vi "draw_extrapolated_lines.vi"(8 "error in (no error)":errorcluster, 11 "TrajectoryMH100122AODRAPS in":refnum<class "TrajectoryMH100122AODRAPS.lvclass">) -> (0 "error out":errorcluster, 3 "TrajectoryMH100122AODRAPS out":refnum<class "TrajectoryMH100122AODRAPS.lvclass">)   [LabVIEW 2010, in "TrajectoryMH100122AODRAPS.lvclass"]
uses:
  TrajectoryMH100122AODRAPS.lvclass
  roi_visualization_cluster.ctl
  common/xcontrols/XImage/XImage/overlays_cluster.ctl
  common/xcontrols/XImage/XImage/XImage.xctl
  TrajectoryMH100122AODRAPS.lvclass/TrajectoryMH100122AODRAPS.ctl
  class_data.vi
  <vilib>/Analysis/1siggen.llb/Ramp Pattern by Samples.vi
  <vilib>/Analysis/NI_AALBase.lvlib
panel:
  in  "zoom":dbl=100.0
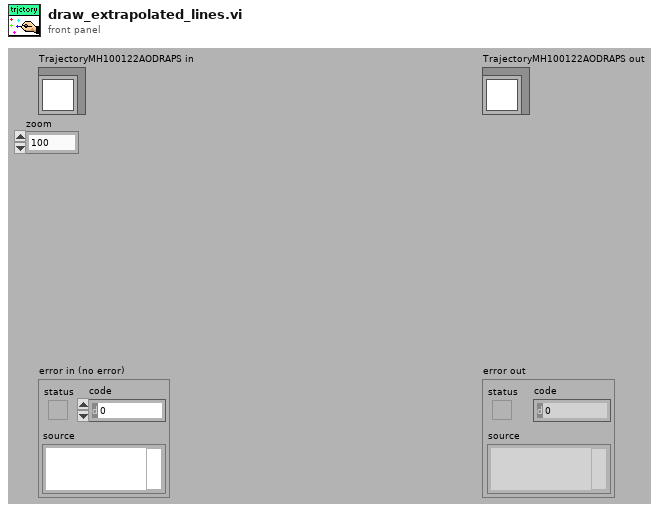
[diagram p1: front panel]
types:
  T1 = typedef "XImage.xctl/overlays_cluster.ctl" = cluster{"overlay array":cluster{i32[][]}[], "overlay name":string, "color (red)":u32, "overlay size":i32, "overlay type":enum16{"crosshair", "circle"}}
  T2 = typedef "TrajectoryMH100122AODRAPS.lvclass/roi_visualization_cluster.ctl" = cluster{"counter":i32, "type":u16, "activation":bool}
  T3 = cluster{"Global Rectangle":i32[], "Contours":cluster{"Contour Type":u32, "ROI Type":u32, "Points":i32[]}[]}[]
  T4 = cluster{"Contour Type":u32, "ROI Type":u32, "Points":i32[]}[]
  T5 = typedef "roi_visualization_cluster.ctl" = cluster{"counter":i32, "type":u16, "activation":bool}
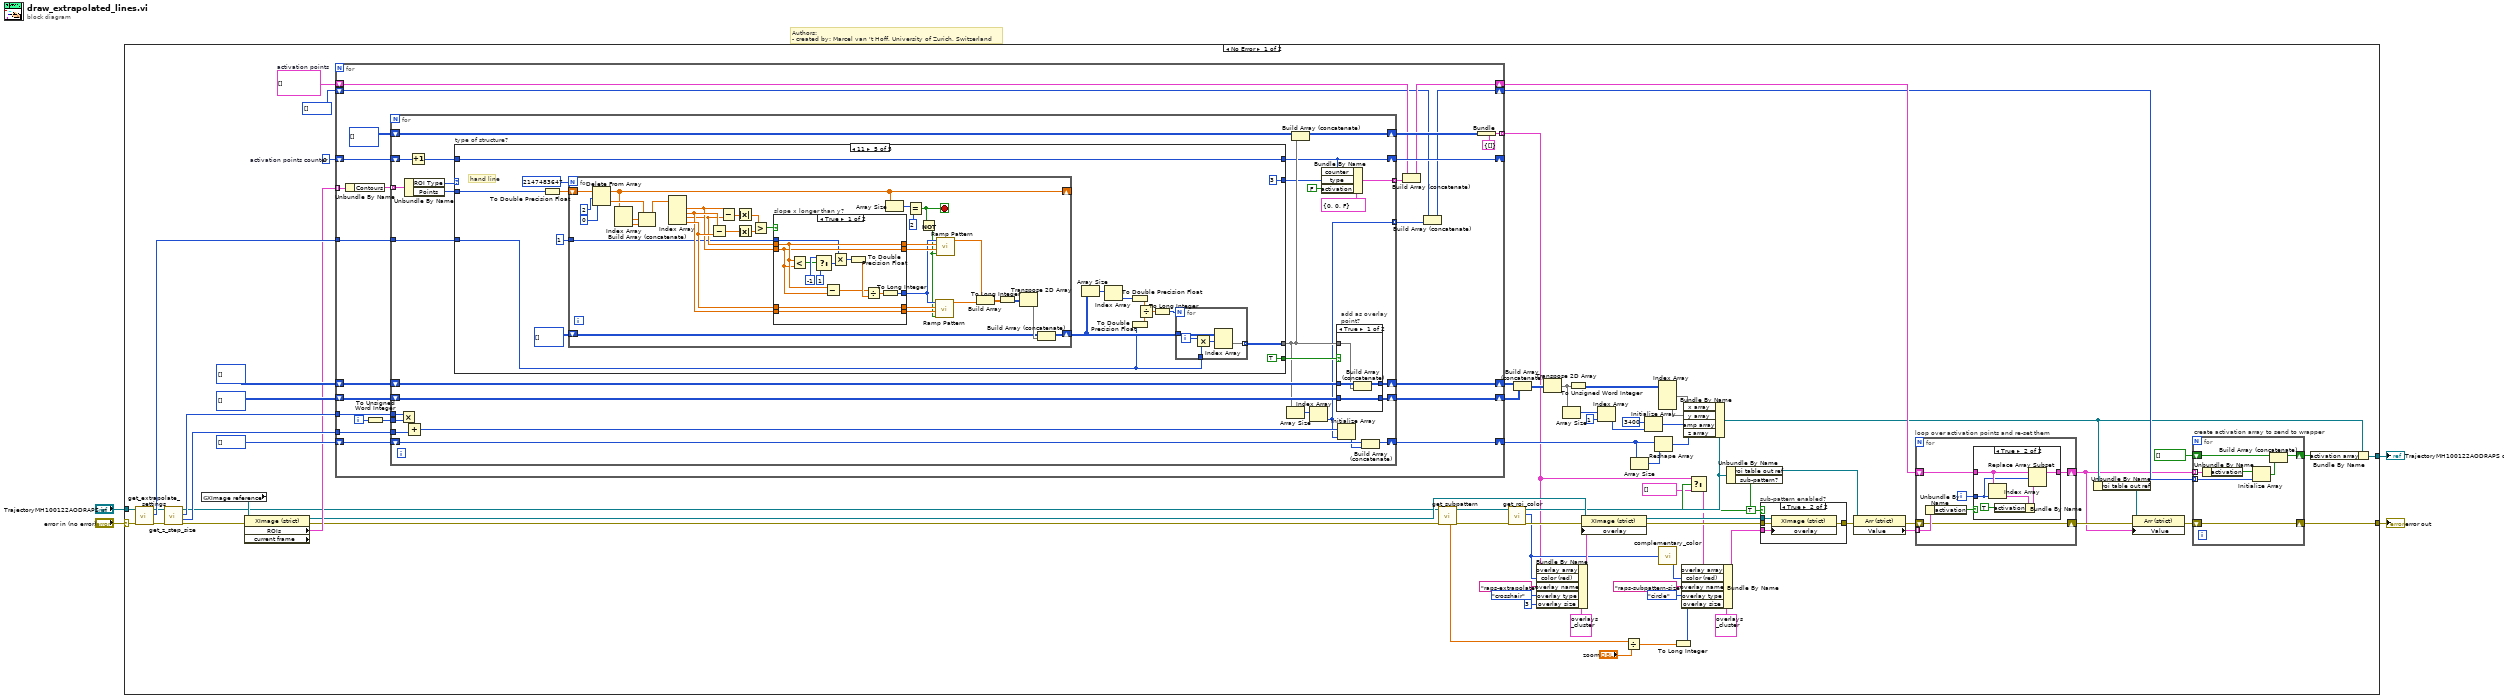
[diagram p0: block diagram]
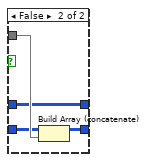
[diagram p4: hidden frame]
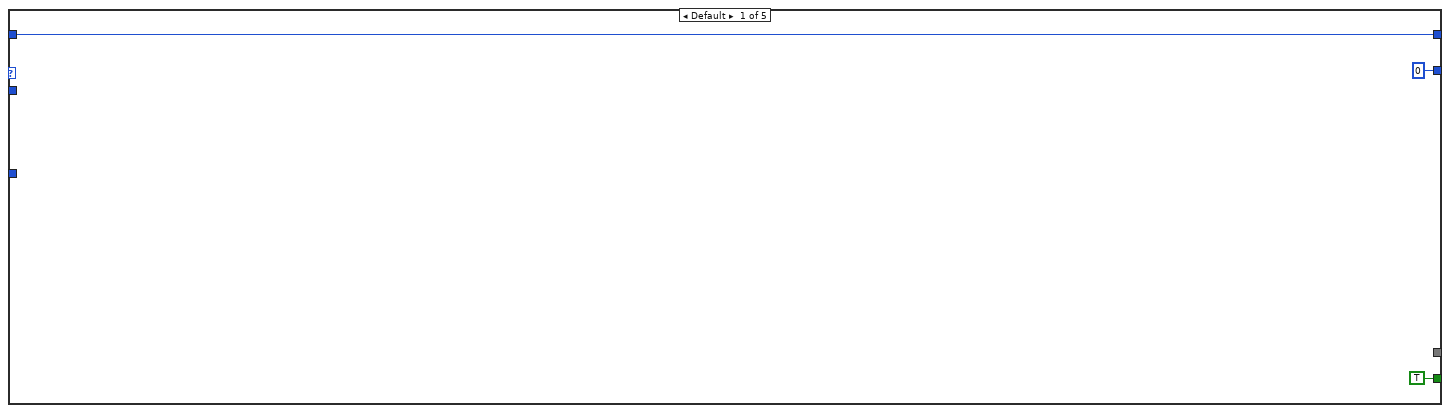
[diagram p5: hidden frame]
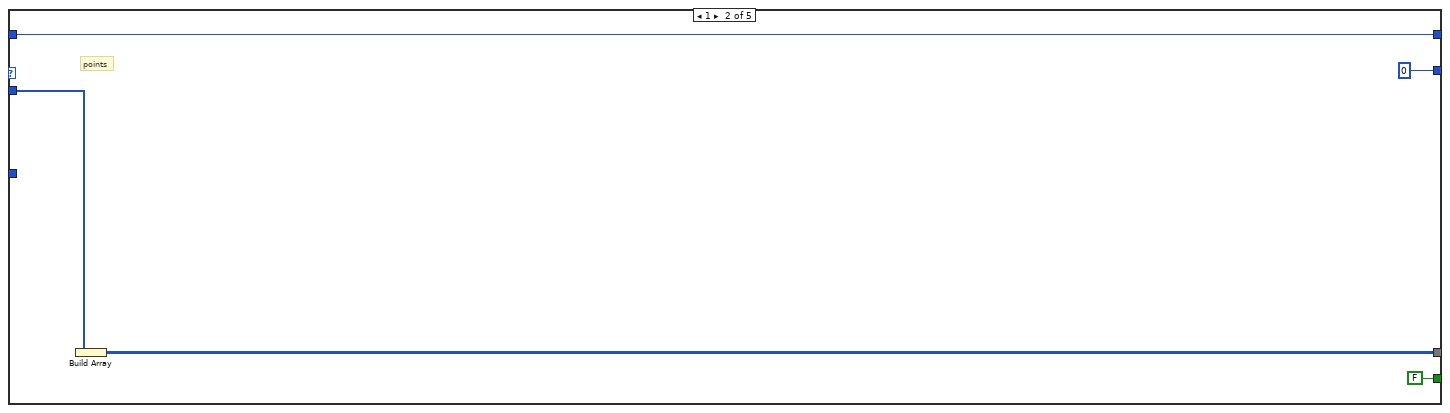
[diagram p6: hidden frame]
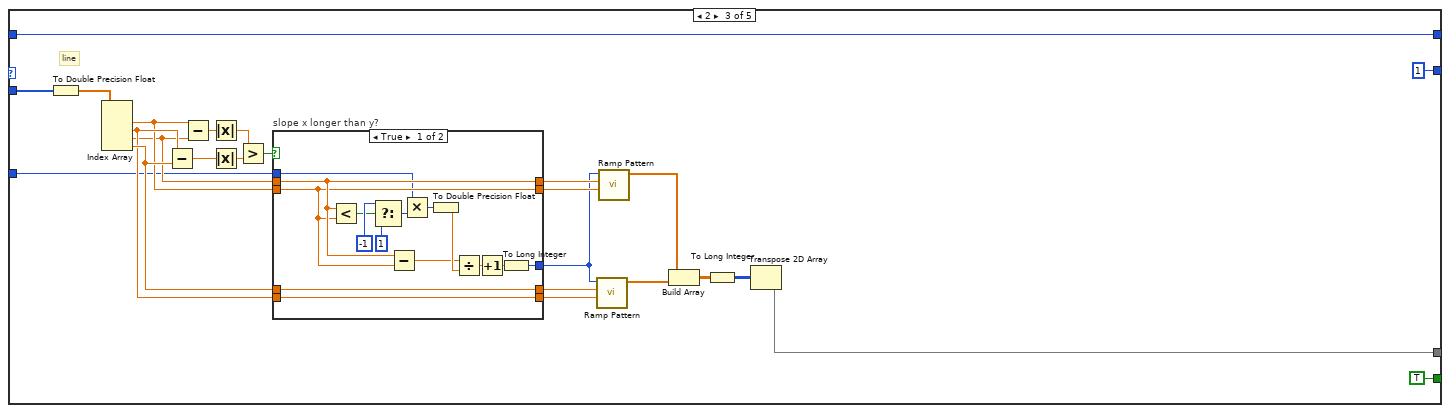
[diagram p7: hidden frame]
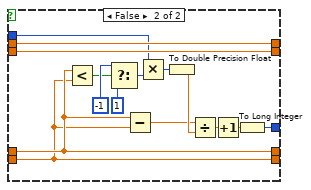
[diagram p8: hidden frame]
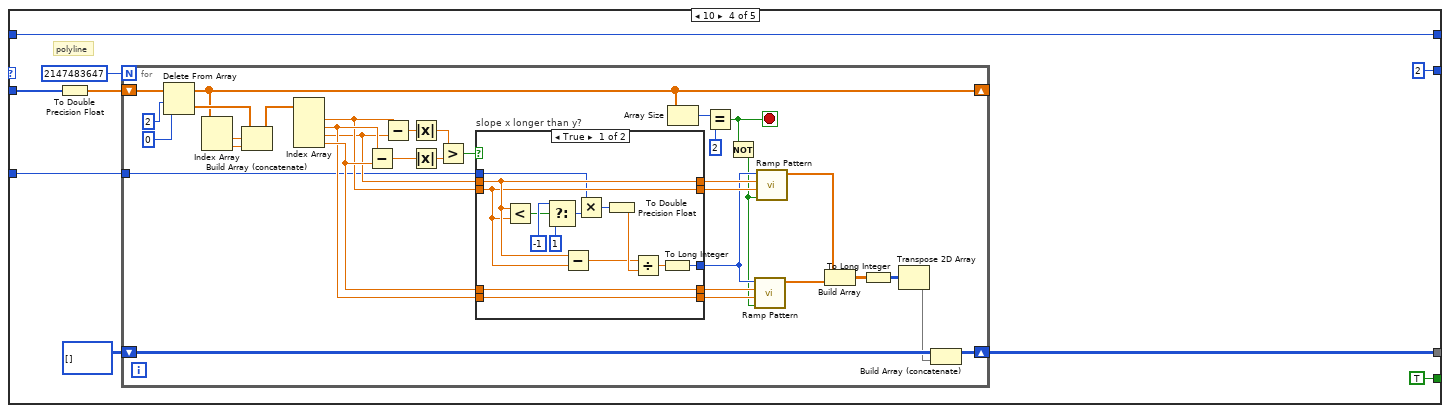
[diagram p9: hidden frame]
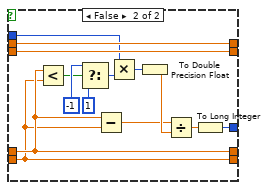
[diagram p10: hidden frame]
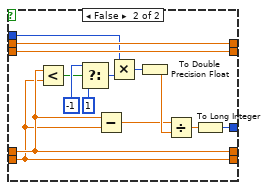
[diagram p11: hidden frame]
diagram:
  # "Authors: \n- created by: Marcel van 't Hoff, University of Zurich, Switzerland"
  n1 = case shown="No Error" "error in (no error)" {
    selector: "error in (no error)" -> [w61 w386]
    tunnel: [w39 w386] -> w3
    tunnel: [w35 w385] -> w1
    tunnel: "TrajectoryMH100122AODRAPS in" -> [w63 w385]
    frame No Error {
      w45 = T2[] []  # activation points
      w46 = 0  # activation points counter
      n2 = call-dynamic "get_extrapolate_settings.vi"("error in (no error)"=w61, "TrajectoryMH100122AODRAPS in"=w63) -> ("error out"=w62:errorcluster, "extrapolate line size"=w78:i32, "TrajectoryMH100122AODRAPS out"=w64:refnum<class "TrajectoryMH100122AODRAPS.lvclass">)  [unwired: 7 in]
      n3 = call-dynamic "get_z_step_size.vi"("error in (no error)"=w62, "TrajectoryMH100122AODRAPS in"=w64) -> ("error out"=w60:errorcluster, "z-offset"=w54:u16, "frame distance"=w59:u16, "TrajectoryMH100122AODRAPS out"=w21:refnum<class "TrajectoryMH100122AODRAPS.lvclass">)  [unwired: 6 in]
      n4 = global read "class_data.vi" "XImage reference"() -> (w51:refnum<vi>)
      n5 = property class="XImage (strict)" props=["ROIs", "current frame"](reference=w51, error in=w60) -> (reference out=w52:refnum<vi>, error out=w19:errorcluster, "ROIs"=w53:T3)  [unwired: 1 out]
      n6 = for {
        tunnel: w53 -> [w129] mode=indexing
        tunnel: w78 -> [w127]
        shift-right: [w118] -> w76
        shift-left: i32[][] [] -> [w126]
        shift-right: [w124] -> w75
        shift-left: i32[][] [] -> [w125]
        tunnel: w59 -> [w123]
        shift-right: [w120] -> w56
        shift-left: u16[] [] -> [w121]
        tunnel: w54 -> [w119]
        tunnel: [w115] -> w11 mode=indexing
        shift-right: [w111] -> _
        shift-left: w46 -> [w112]
        shift-right: [w109] -> w40
        shift-left: w45 -> [w108]
        shift-right: [w107] -> w38
        shift-left: i32[] [] -> [w105]
        i -> [w117]
        n7 = Unbundle By Name(w129) -> ("Contours"=w128:T4)
        n8 = To Unsigned Word Integer(number=w117) -> (unsigned 16bit integer=w122:u16)
        n9 = for {
          tunnel: w128 -> [w158] mode=indexing
          tunnel: w127 -> [w156]
          shift-right: [w146] -> w118
          shift-left: w126 -> [w145]
          shift-right: [w147] -> w124
          shift-left: w125 -> [w144]
          tunnel: w123 -> [w153]
          tunnel: w122 -> [w154]
          shift-right: [w151] -> w120
          shift-left: w121 -> [w152]
          tunnel: w119 -> [w150]
          shift-right: [w142] -> w113
          shift-left: i32[][] [] -> [w143]
          shift-right: [w133] -> w111
          shift-left: w112 -> [w135]
          tunnel: [w132] -> w110 mode=indexing
          tunnel: [w130] -> w106 mode=indexing
          n10 = Multiply(x=w153, y=w154) -> (x*y=w149:u16)
          n11 = Unbundle By Name(w158) -> ("ROI Type"=w157:u32, "Points"=w155:i32[])
          n12 = Add(x=w149, y=w150) -> (x+y=w141:u16)
          n13 = Increment(x=w135) -> (x+1=w134:i32)
          n14 = case "type of structure?" shown="11" w157 {
            tunnel: w156 -> [_ _ w180 w238 w305]
            tunnel: w155 -> [_ w174 w199 w236 w316]
            tunnel: [TRUE FALSE TRUE TRUE TRUE] -> w148
            tunnel: [_ w172 w178 w232 w303] -> w140
            tunnel: [u16 0 u16 0 u16 1 u16 2 u16 3] -> w137
            tunnel: w134 -> [w168 w170 w176 w231 w302]
            tunnel: [w168 w170 w176 w231 w302] -> w133
            frame Default {
            }
            frame 1 {
              # "points"
              n15 = Build Array(w174) -> (w172:i32[][])
            }
            frame 2 {
              # "line"
              n16 = To Double Precision Float(number=w199) -> (double precision float=w191:dbl[])
              n17 = Index Array(array=w191) -> (element #1=w185:dbl, element #2=w187:dbl, element #3=w183:dbl, element #4=w189:dbl)  [unwired: 4 in]
              n18 = Subtract(x=w187, y=w189) -> (x-y=w194:dbl)
              n19 = Subtract(x=w185, y=w183) -> (x-y=w198:dbl)
              n20 = Absolute Value(x=w198) -> (abs(x)=w193:dbl)
              n21 = Absolute Value(x=w194) -> (abs(x)=w192:dbl)
              n22 = Greater?(x=w193, y=w192) -> (0:w190:bool)
              n23 = case "slope x longer than y?" shown="True" w190 {
                tunnel: w183 -> [w204 w221]
                tunnel: w185 -> [w203 w219]
                tunnel: w189 -> [w214 w220]
                tunnel: w187 -> [w213 w218]
                tunnel: [w214 w220] -> w188
                tunnel: [w213 w218] -> w186
                tunnel: [w203 w219] -> w184
                tunnel: [w204 w221] -> w182
                tunnel: w180 -> [w201 w216]
                tunnel: [w202 w217] -> w179
                frame True {
                  n24 = Less?(x=w204, y=w203) -> (x < y?=w205:bool)
                  n25 = Select(t=-1, s=w205, f=1) -> (s? t:f=w208:i32)
                  n26 = Subtract(x=w204, y=w203) -> (x-y=w209:dbl)
                  n27 = Multiply(x=w201, y=w208) -> (x*y=w210:i32)
                  n28 = To Double Precision Float(number=w210) -> (double precision float=w212:dbl)
                  n29 = Divide(x=w209, y=w212) -> (x/y=w211:dbl)
                  n30 = Increment(x=w211) -> (x+1=w200:dbl)
                  n31 = To Long Integer(number=w200) -> (32bit integer=w202:i32)
                }
                frame False {
                  n32 = Less?(x=w220, y=w218) -> (x < y?=w222:bool)
                  n33 = Select(t=-1, s=w222, f=1) -> (s? t:f=w225:i32)
                  n34 = Subtract(x=w220, y=w218) -> (x-y=w226:dbl)
                  n35 = Multiply(x=w216, y=w225) -> (x*y=w227:i32)
                  n36 = To Double Precision Float(number=w227) -> (double precision float=w229:dbl)
                  n37 = Divide(x=w226, y=w229) -> (x/y=w228:dbl)
                  n38 = Increment(x=w228) -> (x+1=w215:dbl)
                  n39 = To Long Integer(number=w215) -> (32bit integer=w217:i32)
                }
              }
              n40 = call-poly <vilib>:"Ramp Pattern.vi"("start"=w186, "end"=w188, "samples"=w179) -> ("Ramp Pattern"=w196:dbl[])  [unwired: 7 in, 1 out]
              n41 = call-poly <vilib>:"Ramp Pattern.vi"("start"=w184, "end"=w182, "samples"=w179) -> ("Ramp Pattern"=w197:dbl[])  [unwired: 7 in, 1 out]
              n42 = Build Array(w197, w196) -> (w195:dbl[][])
              n43 = To Long Integer(number=w195) -> (32bit integer=w181:i32[][])
              n44 = Transpose 2D Array(2D array=w181) -> (transposed array=w178:i32[][])
            }
            frame 10 {
              # "polyline"
              n45 = To Double Precision Float(number=w236) -> (double precision float=w237:dbl[])
              n46 = for {
                N: 2147483647 -> [_]
                tunnel: w238 -> [w256]
                shift-right: [w246] -> _
                shift-left: w237 -> [w253]
                shift-right: [w239] -> w232
                shift-left: i32[][] [] -> [w241]
                stop <- w243 stop-if-true
                n47 = Delete From Array(array=w253, length=2, index=0) -> (deleted portion=w248:dbl[], array with subset deleted=w246:dbl[])
                n48 = Index Array(array=w246) -> (element #1=w250:dbl, element #2=w249:dbl)  [unwired: 2 in]
                n49 = Build Array (concatenate)(w248, w250, w249) -> (w247:dbl[])
                n50 = Index Array(array=w247) -> (element #1=w260:dbl, element #2=w262:dbl, element #3=w258:dbl, element #4=w264:dbl)  [unwired: 4 in]
                n51 = Subtract(x=w262, y=w264) -> (x-y=w268:dbl)
                n52 = Subtract(x=w260, y=w258) -> (x-y=w272:dbl)
                n53 = Absolute Value(x=w272) -> (abs(x)=w267:dbl)
                n54 = Absolute Value(x=w268) -> (abs(x)=w266:dbl)
                n55 = Greater?(x=w267, y=w266) -> (0:w265:bool)
                n56 = case "slope x longer than y?" shown="True" w265 {
                  tunnel: w258 -> [w276 w292]
                  tunnel: w260 -> [w275 w290]
                  tunnel: w264 -> [w286 w291]
                  tunnel: w262 -> [w285 w289]
                  tunnel: [w286 w291] -> w263
                  tunnel: [w285 w289] -> w261
                  tunnel: [w275 w290] -> w259
                  tunnel: [w276 w292] -> w257
                  tunnel: w256 -> [w273 w287]
                  tunnel: [w274 w288] -> w255
                  frame True {
                    n57 = Less?(x=w276, y=w275) -> (x < y?=w277:bool)
                    n58 = Select(t=-1, s=w277, f=1) -> (s? t:f=w280:i32)
                    n59 = Subtract(x=w276, y=w275) -> (x-y=w281:dbl)
                    n60 = Multiply(x=w273, y=w280) -> (x*y=w282:i32)
                    n61 = To Double Precision Float(number=w282) -> (double precision float=w284:dbl)
                    n62 = Divide(x=w281, y=w284) -> (x/y=w283:dbl)
                    n63 = To Long Integer(number=w283) -> (32bit integer=w274:i32)
                  }
                  frame False {
                    n64 = Less?(x=w291, y=w289) -> (x < y?=w293:bool)
                    n65 = Select(t=-1, s=w293, f=1) -> (s? t:f=w296:i32)
                    n66 = Subtract(x=w291, y=w289) -> (x-y=w297:dbl)
                    n67 = Multiply(x=w287, y=w296) -> (x*y=w298:i32)
                    n68 = To Double Precision Float(number=w298) -> (double precision float=w300:dbl)
                    n69 = Divide(x=w297, y=w300) -> (x/y=w299:dbl)
                    n70 = To Long Integer(number=w299) -> (32bit integer=w288:i32)
                  }
                }
                n71 = Array Size(array=w246) -> (size(s)=w245:i32)
                n72 = Equal?(x=w245, y=2) -> (x = y?=w243:bool)
                n73 = Not(x=w243) -> (.not. x?=w242:bool)
                n74 = call-poly <vilib>:"Ramp Pattern.vi"("exclude end?"=w242, "start"=w261, "end"=w263, "samples"=w255) -> ("Ramp Pattern"=w270:dbl[])  [unwired: 6 in, 1 out]
                n75 = call-poly <vilib>:"Ramp Pattern.vi"("exclude end?"=w242, "start"=w259, "end"=w257, "samples"=w255) -> ("Ramp Pattern"=w271:dbl[])  [unwired: 6 in, 1 out]
                n76 = Build Array(w271, w270) -> (w269:dbl[][])
                n77 = To Long Integer(number=w269) -> (32bit integer=w254:i32[][])
                n78 = Transpose 2D Array(2D array=w254) -> (transposed array=w240:i32[][])
                n79 = Build Array (concatenate)(w241, w240) -> (w239:i32[][])
              }
            }
            frame 11 {
              # "hand line"
              n80 = To Double Precision Float(number=w316) -> (double precision float=w315:dbl[])
              n81 = for {
                N: 2147483647 -> [_]
                tunnel: 1 ("extrapolate line size") -> [w339]
                shift-right: [w335] -> w309
                shift-left: i32[][] [] -> [w337]
                shift-right: [w327] -> _
                shift-left: w315 -> [w334]
                stop <- w324 stop-if-true
                n82 = Delete From Array(array=w334, length=2, index=0) -> (deleted portion=w329:dbl[], array with subset deleted=w327:dbl[])
                n83 = Index Array(array=w327) -> (element #1=w331:dbl, element #2=w330:dbl)  [unwired: 2 in]
                n84 = Build Array (concatenate)(w329, w331, w330) -> (w328:dbl[])
                n85 = Index Array(array=w328) -> (element #1=w343:dbl, element #2=w345:dbl, element #3=w341:dbl, element #4=w347:dbl)  [unwired: 4 in]
                n86 = Subtract(x=w345, y=w347) -> (x-y=w351:dbl)
                n87 = Subtract(x=w343, y=w341) -> (x-y=w356:dbl)
                n88 = Absolute Value(x=w356) -> (abs(x)=w350:dbl)
                n89 = Absolute Value(x=w351) -> (abs(x)=w349:dbl)
                n90 = Greater?(x=w350, y=w349) -> (0:w348:bool)
                n91 = case "slope x longer than y?" shown="True" w348 {
                  tunnel: w341 -> [w360 w376]
                  tunnel: w343 -> [w359 w374]
                  tunnel: w347 -> [w370 w375]
                  tunnel: w345 -> [w369 w373]
                  tunnel: [w370 w375] -> w346
                  tunnel: [w369 w373] -> w344
                  tunnel: [w359 w374] -> w342
                  tunnel: [w360 w376] -> w340
                  tunnel: w339 -> [w357 w371]
                  tunnel: [w358 w372] -> w338
                  frame True {
                    n92 = Less?(x=w360, y=w359) -> (x < y?=w361:bool)
                    n93 = Select(t=-1, s=w361, f=1) -> (s? t:f=w364:i32)
                    n94 = Subtract(x=w360, y=w359) -> (x-y=w365:dbl)
                    n95 = Multiply(x=w357, y=w364) -> (x*y=w366:i32)
                    n96 = To Double Precision Float(number=w366) -> (double precision float=w368:dbl)
                    n97 = Divide(x=w365, y=w368) -> (x/y=w367:dbl)
                    n98 = To Long Integer(number=w367) -> (32bit integer=w358:i32)
                  }
                  frame False {
                    n99 = Less?(x=w375, y=w373) -> (x < y?=w377:bool)
                    n100 = Select(t=-1, s=w377, f=1) -> (s? t:f=w380:i32)
                    n101 = Subtract(x=w375, y=w373) -> (x-y=w381:dbl)
                    n102 = Multiply(x=w371, y=w380) -> (x*y=w382:i32)
                    n103 = To Double Precision Float(number=w382) -> (double precision float=w384:dbl)
                    n104 = Divide(x=w381, y=w384) -> (x/y=w383:dbl)
                    n105 = To Long Integer(number=w383) -> (32bit integer=w372:i32)
                  }
                }
                n106 = Array Size(array=w327) -> (size(s)=w326:i32)
                n107 = Equal?(x=w326, y=2) -> (x = y?=w324:bool)
                n108 = Not(x=w324) -> (.not. x?=w323:bool)
                n109 = call-poly <vilib>:"Ramp Pattern.vi"("exclude end?"=w323, "start"=w344, "end"=w346, "samples"=w338) -> ("Ramp Pattern"=w354:dbl[])  [unwired: 6 in, 1 out]
                n110 = call-poly <vilib>:"Ramp Pattern.vi"("exclude end?"=w323, "start"=w342, "end"=w340, "samples"=w338) -> ("Ramp Pattern"=w355:dbl[])  [unwired: 6 in, 1 out]
                n111 = Build Array(w355, w354) -> (w353:dbl[][])
                n112 = To Long Integer(number=w353) -> (32bit integer=w336:i32[][])
                n113 = Transpose 2D Array(2D array=w336) -> (transposed array=w352:i32[][])
                n114 = Build Array (concatenate)(w337, w352) -> (w335:i32[][])
              }
              n115 = Array Size(array=w309) -> (size(s)=w313:i32[])
              n116 = Index Array(array=w313) -> (element=w312:i32)  [unwired: 1 in]
              n117 = To Double Precision Float(number=w312) -> (double precision float=w307:dbl)
              n118 = To Double Precision Float(number=w305) -> (double precision float=w306:dbl)
              n119 = Divide(x=w307, y=w306) -> (x/y=w311:dbl)
              n120 = To Long Integer(number=w311) -> (32bit integer=w310:i32)
              n121 = for {
                N: w310 -> [_]
                tunnel: w309 -> [w322]
                tunnel: w305 -> [w320]
                tunnel: [w319] -> w303 mode=indexing
                i -> [w321]
                n122 = Multiply(x=w321, y=w320) -> (x*y=w318:i32)
                n123 = Index Array(array=w322, index (row)=w318) -> (element=w319:i32[])  [unwired: 1 in]
              }
            }
          }
          n124 = Array Size(array=w140) -> (size(s)=w131:i32[])
          n125 = Build Array (concatenate)(w143, w140) -> (w142:i32[][])
          n126 = Index Array(array=w131) -> (element=w130:i32)  [unwired: 1 in]
          n127 = Bundle By Name(cluster=T2 {"counter"=0, "type"=0, "activation"=FALSE} ("System Cluster"), "counter"=w133, "type"=w137, "activation"=FALSE) -> (w132:T2)
          n128 = case "add as overlay \npoint?" shown="True" w148 {
            tunnel: [w161 w163] -> w146
            tunnel: w145 -> [w162 w163]
            tunnel: [w159 w164] -> w147
            tunnel: w144 -> [w159 w165]
            tunnel: w140 -> [w160 w166]
            frame True {
              n129 = Build Array (concatenate)(w162, w160) -> (w161:i32[][])
            }
            frame False {
              n130 = Build Array (concatenate)(w165, w166) -> (w164:i32[][])
            }
          }
          n131 = Initialize Array(w141, w130) -> (w139:u16[])
          n132 = Build Array (concatenate)(w152, w139) -> (w151:u16[])
        }
        n133 = Build Array (concatenate)(w108, w110) -> (w109:T2[])
        n134 = Build Array (concatenate)(w105, w106) -> (w107:i32[])
        n135 = Bundle(cluster=cluster{i32[][]} {[]}, w113) -> (w115:cluster{i32[][]})
      }
      n136 = call-dynamic "get_subpattern.vi"("error in (no error)"=w19, "TrajectoryMH100122AODRAPS in"=w21) -> ("error out"=w18:errorcluster, "TrajectoryMH100122AODRAPS out"=w20:refnum<class "TrajectoryMH100122AODRAPS.lvclass">, "diameter"=w6:dbl)  [unwired: 4 in, 3 out]
      n137 = call-dynamic "get_roi_color.vi"("error in (no error)"=w18, "TrajectoryMH100122AODRAPS in"=w20) -> ("error out"=w48:errorcluster, "ROI color"=w23:u32, "TrajectoryMH100122AODRAPS out"=w13:refnum<class "TrajectoryMH100122AODRAPS.lvclass">)  [unwired: 7 in]
      n138 = Build Array (concatenate)(w76, w75) -> (w74:i32[][])
      n139 = Bundle By Name(cluster=T1 {"overlay array"=[], "overlay name"="", "color (red)"=16711680, "overlay size"=0, "overlay type"=enum."crosshair"} ("Overlay"), "overlay array"=w11, "color (red)"=w23, "overlay name"="raps-extrapolate", "overlay type"=enum16{"crosshair", "circle"}."crosshair", "overlay size"=3 ("cross hair size")) -> (w47:T1)
      n140 = Transpose 2D Array(2D array=w74) -> (transposed array=w70:i32[][])
      n141 = Array Size(array=w70) -> (size(s)=w69:i32[])
      n142 = To Unsigned Word Integer(number=w70) -> (unsigned 16bit integer=w71:u16[][])
      n143 = property class="XImage (strict)"(reference=w52, error in=w48, "overlay"=w47) -> (reference out=w29:refnum<vi>, error out=w28:errorcluster)
      n144 = Index Array(array=w69, index=1) -> (element=w65:i32)
      n145 = Divide(x=w6, y="zoom") -> (x/y=w5:dbl)
      n146 = Array Size(array=w56) -> (size(s)=w55:i32)
      n147 = Initialize Array(u16 3400, w65) -> (w66:u16[])
      n148 = Reshape Array(w56, w55) -> (w58:u16[])
      n149 = Index Array(array=w71) -> (element #1=w73:u16[], element #2=w72:u16[])  [unwired: 4 in]
      n150 = call "complementary_color.vi"("color in"=w23) -> ("complementary color out"=w22:u32)
      n151 = To Long Integer(number=w5) -> (32bit integer=w14:i32)
      n152 = Bundle By Name(cluster=w13, "x array"=w73, "y array"=w72, "amp array"=w66, "z array"=w58) -> (w34:refnum<class "TrajectoryMH100122AODRAPS.lvclass">)
      n153 = Unbundle By Name(w13) -> ("roi table out ref"=w41:refnum<vi>, "sub-pattern?"=w12:bool)
      n154 = Select(t=w11, s=w12, f=cluster{i32[][]}[] []) -> (s? t:f=w9:cluster{i32[][]}[])
      n155 = Bundle By Name(cluster=T1 {"overlay array"=[], "overlay name"="", "color (red)"=16711680, "overlay size"=0, "overlay type"=enum."crosshair"} ("Overlay"), "overlay array"=w9, "color (red)"=w22, "overlay name"="raps-subpattern-size", "overlay type"=enum16{"crosshair", "circle"}."circle", "overlay size"=w14) -> (w24:T1)
      n156 = case "sub-pattern enabled?" shown="True" TRUE {
        tunnel: w29 -> [_ w84]
        tunnel: w28 -> [w80 w83]
        tunnel: [w80 w82] -> w27
        tunnel: w24 -> [_ w81]
        frame False {
        }
        frame True {
          n157 = property class="XImage (strict)"(reference=w84, error in=w83, "overlay"=w81) -> (error out=w82:errorcluster)  [unwired: 1 out]
        }
      }
      n158 = property class="Arr (strict)"(reference=w41, error in=w27) -> (error out=w43:errorcluster, "Value"=w42:T5[])  [unwired: 1 out]
      n159 = for "loop over activation points and re-set them" {
        tunnel: w42 -> [w97] mode=indexing
        shift-right: [w93] -> w30
        shift-left: w40 -> [w96]
        shift-right: [w92] -> w32
        shift-left: w43 -> [w92]
        i -> [w95]
        n160 = Unbundle By Name(w97) -> ("activation"=w94:bool)
        n161 = case shown="True" w94 {
          tunnel: w96 -> [w98 w104]
          tunnel: w95 -> [_ w103]
          tunnel: [w98 w99] -> w93
          frame False {
          }
          frame True {
            n162 = Index Array(array=w104, index=w103) -> (element=w102:T2)
            n163 = Bundle By Name(cluster=w102, "activation"=TRUE) -> (w100:T2)
            n164 = Replace Array Subset(array=w104, new element=w100, index=w103) -> (w99:T2[])
          }
        }
      }
      n165 = Unbundle By Name(w34) -> ("roi table out ref"=w33:refnum<vi>)
      n166 = property class="Arr (strict)"(reference=w33, error in=w32, "Value"=w30) -> (error out=w31:errorcluster)  [unwired: 1 out]
      n167 = for "create activation array to send to wrapper" {
        tunnel: w30 -> [w91] mode=indexing
        shift-right: [w90] -> w39
        shift-left: w31 -> [w90]
        tunnel: w38 -> [w88] mode=indexing
        shift-right: [w86] -> w36
        shift-left: bool[] [] -> [w87]
        n168 = Unbundle By Name(w91) -> ("activation"=w89:bool)
        n169 = Initialize Array(w89, w88) -> (w85:bool[])
        n170 = Build Array (concatenate)(w87, w85) -> (w86:bool[])
      }
      n171 = Bundle By Name(cluster=w34, "activation array"=w36) -> (w35:refnum<class "TrajectoryMH100122AODRAPS.lvclass">)
    }
    frame Error {
    }
  }
  "error out" <- w3
  "TrajectoryMH100122AODRAPS out" <- w1
